vi "HFRR ADV v04 new software.vi"() -> ()   [LabVIEW 2025] (continued)
        n807 = local write "CAMERA ROI MAX TEMP"(TRUE ("CAMERA ROI MAX TEMP")) -> ()
      }
      frame "About" {
        n808 = local read "LIVE FEED MIN TEMP"() -> (w1181:bool)
        n809 = local write "LIVE FEED MAX TEMP"(TRUE ("LIVE FEED MAX TEMP")) -> ()
        n810 = local read "CAMERA ROI MIN TEMP"() -> (w1180:bool)
        n811 = case shown="True" w1181 {
          selector: w1181 -> [_ w1188]
          frame False {
          }
          frame True {
            n812 = Not(x=w1188) -> (.not. x?=w1187:bool)
            n813 = local write "LIVE FEED MIN TEMP"(w1187) -> ()
            n814 = call "CAMERA LIVE FEED FGV.vi"("Enum - Menu"=CAMERA_LIVE_FEED_ENUM."CAMERA MINIMIZE") -> ()  [unwired: 9 in, 2 out]
          }
        }
        n815 = case shown="True" w1180 {
          selector: w1180 -> [_ w1185]
          frame False {
          }
          frame True {
            n816 = Not(x=w1185) -> (.not. x?=w1184:bool)
            n817 = local write "CAMERA ROI MIN TEMP"(w1184) -> ()
            n818 = call "IMAGE ANALYSIS.vi"("Enum"=POST_ANALYSIS_ENUM."MINIMIZE UI") -> ()  [unwired: 9 in, 2 out]
          }
        }
        n819 = local write "CAMERA ROI MAX TEMP"(TRUE ("CAMERA ROI MIN TEMP")) -> ()
      }
      frame "Advance" {
        n820 = local read "LIVE FEED MIN TEMP"() -> (w1191:bool)
        n821 = local write "LIVE FEED MAX TEMP"(TRUE ("LIVE FEED MAX TEMP")) -> ()
        n822 = local read "CAMERA ROI MIN TEMP"() -> (w1189:bool)
        n823 = case shown="True" w1191 {
          selector: w1191 -> [_ w1198]
          frame False {
          }
          frame True {
            n824 = Not(x=w1198) -> (.not. x?=w1197:bool)
            n825 = local write "LIVE FEED MIN TEMP"(w1197) -> ()
            n826 = call "CAMERA LIVE FEED FGV.vi"("Enum - Menu"=CAMERA_LIVE_FEED_ENUM."CAMERA MINIMIZE") -> ()  [unwired: 9 in, 2 out]
          }
        }
        n827 = local write "CAMERA ROI MAX TEMP"(TRUE ("CAMERA ROI MAX TEMP")) -> ()
        n828 = case shown="True" w1189 {
          selector: w1189 -> [_ w1195]
          frame False {
          }
          frame True {
            n829 = Not(x=w1195) -> (.not. x?=w1194:bool)
            n830 = local write "CAMERA ROI MIN TEMP"(w1194) -> ()
            n831 = call "IMAGE ANALYSIS.vi"("Enum"=POST_ANALYSIS_ENUM."MINIMIZE UI") -> ()  [unwired: 9 in, 2 out]
          }
        }
      }
      frame "Mooha" {
        n832 = local read "LIVE FEED MIN TEMP"() -> (w1201:bool)
        n833 = local write "LIVE FEED MAX TEMP"(TRUE ("LIVE FEED MAX TEMP")) -> ()
        n834 = local read "CAMERA ROI MIN TEMP"() -> (w1199:bool)
        n835 = case shown="True" w1201 {
          selector: w1201 -> [_ w1208]
          frame False {
          }
          frame True {
            n836 = Not(x=w1208) -> (.not. x?=w1207:bool)
            n837 = local write "LIVE FEED MIN TEMP"(w1207) -> ()
            n838 = call "CAMERA LIVE FEED FGV.vi"("Enum - Menu"=CAMERA_LIVE_FEED_ENUM."CAMERA MINIMIZE") -> ()  [unwired: 9 in, 2 out]
          }
        }
        n839 = local write "CAMERA ROI MAX TEMP"(TRUE ("CAMERA ROI MAX TEMP")) -> ()
        n840 = case shown="True" w1199 {
          selector: w1199 -> [_ w1205]
          frame False {
          }
          frame True {
            n841 = Not(x=w1205) -> (.not. x?=w1204:bool)
            n842 = local write "CAMERA ROI MIN TEMP"(w1204) -> ()
            n843 = call "IMAGE ANALYSIS.vi"("Enum"=POST_ANALYSIS_ENUM."MINIMIZE UI") -> ()  [unwired: 9 in, 2 out]
          }
        }
      }
    }
    n844 = local read "Auto Start Test"() -> (w950:bool)
    n845 = case shown="True" "sign in temp" {
      frame False {
      }
      frame True {
        w987 = 1 ("y")
        n846 = local read "USERNAME"() -> (w993:string)
        n847 = local read "USER ID"() -> (w990:string)
        n848 = call <vilib>:"Trim Whitespace.vi"("string"=w993) -> ("trimmed string"=w992:string)  [unwired: 1 in]
        n849 = call <vilib>:"Trim Whitespace.vi"("string"=w990) -> ("trimmed string"=w991:string)  [unwired: 1 in]
        n850 = String Length(string=w992) -> (length=w989:i32)
        n851 = String Length(string=w991) -> (length=w988:i32)
        n852 = Greater?(x=w989, y=w987) -> (0:w986:bool)
        n853 = Greater?(x=w988, y=w987) -> (0:w985:bool)
        n854 = And(x=w986, y=w985) -> (x .and. y?=w984:bool)
        n855 = case shown="True" w984 {
          frame False {
            n856 = property on="Sign In" class="Bool (strict)"("DisabledEnum"=T13."Disabled" ("Disabled")) -> ()  [unwired: 2 in, 2 out]
          }
          frame True {
            n857 = property on="Sign In" class="Bool (strict)"("DisabledEnum"=T13."Enabled" ("Disabled")) -> ()  [unwired: 2 in, 2 out]
          }
        }
      }
    }
    n858 = local read "Air Temperature"() -> (w967:bool)
    n859 = local read "Coefficient Of Friction"() -> (w968:bool)
    n860 = case shown="False" w950 {
      frame False {
        n861 = local read "Auto stop temp"() -> (w981:bool)
        n862 = case shown="True" w981 {
          frame False {
          }
          frame True {
            n863 = local write "Auto Start Temp"(FALSE ("Auto Start Temp")) -> ()
          }
        }
      }
      frame True {
        "Auto stop temp" <- TRUE ("Auto stop temp")
      }
    }
    n864 = local read "Humidity"() -> (w966:bool)
    n865 = case shown="\"HOME\"" w978 {
      frame "HOME" {
        n866 = local write "main tab sub"(enum32{"Page 1", "Page 2"}."Page 1" ("main tab sub")) -> ()
      }
      frame Default {
        n867 = local write "main tab sub"(enum32{"Page 1", "Page 2"}."Page 2" ("main tab sub")) -> ()
      }
    }
    n868 = case shown="True" w977 {
      selector: w977 -> [_ w1313]
      frame False {
      }
      frame True {
        n869 = Not(x=w1313) -> (.not. x?=w1312:bool)
        n870 = local write "Sign In"(w1312) -> ()
        n871 = local write "Main Dashboard Buttons"(T1."Test Setup" ("Main Dashboard Buttons")) -> ()
      }
    }
    n872 = case shown="\"Numeric Display\", Default" "Num/Graph" {
      frame "Numeric Display", Default {
        n873 = property on="Single/Multiple" class="RadioBtnsControl (strict)"("Visible"=FALSE) -> ()  [unwired: 2 in, 2 out]
        n874 = property on="Single - Graph" class="Ring (strict)"("Visible"=FALSE) -> ()  [unwired: 2 in, 2 out]
        n875 = local write "Main Tab Display"(T4."Dashboard 1" ("Main Tab Display")) -> ()
      }
      frame "Graph Display" {
        n876 = property on="Single/Multiple" class="RadioBtnsControl (strict)"("Visible"=TRUE) -> ()  [unwired: 2 in, 2 out]
        n877 = case shown="\"Multiple\"" "Single/Multiple" {
          frame "Single ", Default {
            n878 = property on="Single - Graph" class="Ring (strict)"("Visible"=TRUE) -> ()  [unwired: 2 in, 2 out]
            n879 = local write "Main Tab Display"(T4."Dashboard 3" ("Main Tab Display")) -> ()
          }
          frame "Multiple" {
            n880 = property on="Single - Graph" class="Ring (strict)"("Visible"=FALSE) -> ()  [unwired: 2 in, 2 out]
            n881 = local write "Main Tab Display"(T4."Dashboard 2" ("Main Tab Display")) -> ()
          }
        }
      }
    }
    n882 = local read "Stroke"() -> (w965:bool)
    n883 = local read "USERNAME"() -> (w971:string)
    n884 = local read "USER ID"() -> (w970:string)
    n885 = case shown="True" w968 {
      selector: w968 -> [_ w1248]
      frame False {
      }
      frame True {
        n886 = Not(x=w1248) -> (.not. x?=w1247:bool)
        n887 = local write "Coefficient Of Friction"(w1247) -> ()
        n888 = local write "Tab Control 2"(T6."Coefficient Of Friction" ("Tab Control 2")) -> ()
      }
    }
    n889 = case shown="True" w967 {
      selector: w967 -> [_ w1245]
      frame False {
      }
      frame True {
        n890 = Not(x=w1245) -> (.not. x?=w1243:bool)
        n891 = local write "Air Temperature"(w1243) -> ()
        n892 = local write "Tab Control 2"(T6."Air Temperature" ("Tab Control 2")) -> ()
      }
    }
    n893 = local write "Operator ID"(w970) -> ()
    n894 = case shown="True" w965 {
      selector: w965 -> [_ w1239]
      frame False {
      }
      frame True {
        n895 = Not(x=w1239) -> (.not. x?=w1237:bool)
        n896 = local write "Stroke"(w1237) -> ()
        n897 = local write "Tab Control 2"(T6."Stroke" ("Tab Control 2")) -> ()
      }
    }
    n898 = local write "tested by"(w971) -> ()
    n899 = case shown="True" w966 {
      selector: w966 -> [_ w1242]
      frame False {
      }
      frame True {
        n900 = Not(x=w1242) -> (.not. x?=w1240:bool)
        n901 = local write "Humidity"(w1240) -> ()
        n902 = local write "Tab Control 2"(T6."Humidity" ("Tab Control 2")) -> ()
      }
    }
    n903 = case shown="\"Advance\"" "Main Dashboard Buttons" {
      tunnel: [T2."HOME" ("Main Tab") T2."Test Setup" ("Main Tab") T2."Acquire" ("Main Tab") T2."Adv Scar" ("Main Tab") T2."Adv Scar Report" ("Main Tab") T2."Compare Files" ("Main Tab") T2."About" ("Main Tab") T2."Advance" ("Main Tab")] -> w975
      frame "Home", Default {
      }
      frame "Test Setup" {
      }
      frame "Dashboard" {
      }
      frame "Imaging" {
      }
      frame "Report" {
      }
      frame "Analysis" {
      }
      frame "About" {
      }
      frame "Advance" {
      }
    }
    n904 = Wait (ms)(milliseconds to wait=u32 100) -> ()  [unwired: 1 out]
    n905 = local read "Main Tab Display"() -> (w969:T4)
    n906 = local write "Main Tab"(w975) -> ()
    n907 = case shown="\"Dashboard 3\"" w969 {
      frame "Dashboard 1", Default {
        n908 = property on="Reset Graph" class="Bool (strict)"("Visible"=FALSE) -> ()  [unwired: 2 in, 2 out]
      }
      frame "Dashboard 2" {
        n909 = property on="Reset Graph" class="Bool (strict)"("Visible"=TRUE) -> ()  [unwired: 2 in, 2 out]
      }
      frame "Dashboard 3" {
        n910 = property on="Reset Graph" class="Bool (strict)"("Visible"=TRUE) -> ()  [unwired: 2 in, 2 out]
      }
    }
    n911 = local read "SCAR MEASURMENT"() -> (w957:enum32{"Auto Scar", "Manual Scar"})
    n912 = local read "Humidity"() -> (w972:bool)
    n913 = local read "Cap Live Image"() -> (w954:bool)
    n914 = local read "Sample Temperature"() -> (w964:bool)
    n915 = local read "Air Temp vs Humidity"() -> (w962:bool)
    n916 = local read "Frequency"() -> (w963:bool)
    n917 = case shown="False" w972 {
      frame False {
        n918 = local write "Humidity On Command"(TRUE ("Humidity On Command")) -> ()
        n919 = case shown="True" "Humidity Off Command" {
          selector: "Humidity Off Command" -> [_ w1255]
          frame False {
          }
          frame True {
            n920 = stacked-sequence {
              frame #0 {
                n921 = local read "WriteHumidity"() -> (w1257:string[])
                n922 = Insert Into Array(array=w1257, new element="R;1" ("new element/subarray")) -> (w1258:string[])  [unwired: 1 in]
                n923 = local write "WriteHumidity"(w1258) -> ()
              }
              frame #1 {
                n924 = Wait (ms)(milliseconds to wait=u32 2000) -> ()  [unwired: 1 out]
              }
              frame #2 {
                n925 = local read "EVENT LOG"() -> (w1264:string)
                n926 = local read "WriteHumidity"() -> (w1261:string[])
                n927 = call "Event Log.vi"("Content"="Humidity Control Off" ("string"), "EVENT LOG"=w1264) -> ("EVENT LOG"=w1265:string)  [unwired: 8 in, 1 out]
                n928 = local write "EVENT LOG"(w1265) -> ()
                n929 = Insert Into Array(array=w1261, new element="R;1" ("new element/subarray")) -> (w1262:string[])  [unwired: 1 in]
                n930 = local write "WriteHumidity"(w1262) -> ()
              }
            }
            n931 = Not(x=w1255) -> (.not. x?=w1254:bool)
            n932 = local write "Humidity Off Command"(w1254) -> ()
          }
        }
      }
      frame True {
        n933 = local write "Humidity Off Command"(TRUE ("Humidity Off Command")) -> ()
        n934 = case shown="False" "Humidity On Command" {
          selector: "Humidity On Command" -> [_ w1269]
          frame False {
          }
          frame True {
            n935 = stacked-sequence {
              frame #0 {
                n936 = local read "Set Rh"() -> (w1275:dbl)
                n937 = Number To Fractional String(number=w1275, precision (6)=i16 2) -> (F-format string=w1276:string)  [unwired: 2 in]
                n938 = local read "WriteHumidity"() -> (w1273:string[])
                n939 = Concatenate Strings("M;" ("new element/subarray"), w1276) -> (w1274:string)
                n940 = Insert Into Array(array=w1273, new element=w1274) -> (w1272:string[])  [unwired: 1 in]
                n941 = local write "WriteHumidity"(w1272) -> ()
              }
              frame #1 {
                n942 = Wait (ms)(milliseconds to wait=u32 1500) -> ()  [unwired: 1 out]
              }
              frame #2 {
                (unwired) "% RH" ("string")
                (unwired) i16 2 ("precision (6)")
                (unwired) "M;" ("new element/subarray")
                n943 = local read "Set Rh"() -> (w1283:dbl)
                n944 = Number To Fractional String(number=w1283, precision (6)=i16 2) -> (F-format string=w1280:string)  [unwired: 2 in]
                n945 = local read "WriteHumidity"() -> (w1285:string[])
                n946 = Concatenate Strings("M;" ("new element/subarray"), w1280) -> (w1284:string)
                n947 = Concatenate Strings("Humidity Set to : " ("string"), w1280, "% RH" ("string")) -> (w1278:string)
                n948 = Insert Into Array(array=w1285, new element=w1284) -> (w1286:string[])  [unwired: 1 in]
                n949 = disable-structure shown="Enabled" {
                  frame Enabled {
                    n950 = local read "EVENT LOG"() -> (w1289:string)
                    n951 = call "Event Log.vi"("Content"="Humidity Control On", "EVENT LOG"=w1289) -> ("EVENT LOG"=w1290:string)  [unwired: 8 in, 1 out]
                    n952 = local write "EVENT LOG"(w1290) -> ()
                  }
                  frame Disabled {
                  }
                }
                n953 = disable-structure shown="Enabled" {
                  disable-tunnel: w1278 -> [_ _]
                  frame Enabled {
                    n954 = local read "EVENT LOG"() -> (w1292:string)
                    n955 = call "Event Log.vi"("Content"="Humidity Control On", "EVENT LOG"=w1292) -> ("EVENT LOG"=w1293:string)  [unwired: 8 in, 1 out]
                    n956 = local write "EVENT LOG"(w1293) -> ()
                  }
                  frame Disabled {
                  }
                }
                n957 = local write "WriteHumidity"(w1286) -> ()
              }
            }
            n958 = Not(x=w1269) -> (.not. x?=w1268:bool)
            n959 = local write "Humidity On Command"(w1268) -> ()
          }
        }
      }
    }
    n960 = Equal?(x=w957, y=enum32{"Auto Scar", "Manual Scar"}."Auto Scar" ("SCAR MEASURMENT")) -> (x = y?=w953:bool)
    n961 = local read "TEST STANDARD"() -> (w960:T3)
    n962 = And(x=w954, y=w953) -> (x .and. y?=w955:bool)
    n963 = case shown="True" w955 {
      selector: w955 -> [_ w1054]
      tunnel: errorcluster {"status"=FALSE, "code"=0, "source"=""} ("error in (no error) 3") -> [_ w1055]
      frame False {
      }
      frame True {
        n964 = stacked-sequence {
          tunnel: w1055 -> [_ _ _ _ _ _ _ w1103]
          tunnel: w1054 -> [_ _ _ _ _ w1084 _ _]
          frame #0 {
            n965 = call "CAMERA LIVE FEED FGV.vi"("Enum - Menu"=CAMERA_LIVE_FEED_ENUM."CAMERA MINIMIZE") -> ()  [unwired: 9 in, 2 out]
          }
          frame #1 {
            n966 = property on="Auto Scar Check  2" class="Clust (strict)"("Visible"=TRUE) -> ()  [unwired: 2 in, 2 out]
          }
          frame #2 {
            n967 = String To Path(string="C:\\LAB-IQ\\Image Calibrate v01.dcf") -> (path=w1060:path)
            n968 = Open/Create/Replace File ("Open File")(file path (use dialog)=w1060) -> (refnum out=w1061:refnum<file>)  [unwired: 5 in, 2 out]
            n969 = for {
              N: 4 -> [_]
              tunnel: w1061 -> [w1067]
              i -> [w1063]
              n970 = Read from Text File ("Read File")(file (use dialog)=w1067) -> (text=w1068:string)  [unwired: 3 in, 3 out]
              n971 = String Subset(string=w1068, offset (0)=6, length (rest)=10 ("length (rest)")) -> (substring=w1064:string)
              n972 = Fract/Exp String To Number(string=w1064) -> (number=w1062:dbl)  [unwired: 3 in, 1 out]
              n973 = case shown="0" w1063 {
                tunnel: w1062 -> [w1069 w1070 _ w1071 _]
                frame 0 {
                  "5x Gain" <- w1069
                }
                frame 1 {
                  "10x Gain" <- w1070
                }
                frame 2 {
                }
                frame 3 {
                  "100x gain" <- w1071
                }
                frame 4, Default {
                }
              }
            }
          }
          frame #3 {
            n974 = local read "FILE 3"() -> (w1077:string)
            n975 = call <vilib>:"Trim Whitespace.vi"("string"="C:\\LAB-IQ\\images\\") -> ("trimmed string"=w1079:string)  [unwired: 1 in]
            n976 = String To Path(string=w1079) -> (path=w1078:path)
            n977 = Concatenate Strings(w1077, ".png" ("string")) -> (w1076:string)
            n978 = Build Path(base path=w1078, name or relative path=w1076) -> (appended path=w1074:path)
            "Image path" <- w1074
            n979 = Path To String(path=w1074) -> (string=w1073:string)
            n980 = call "CAMERA LIVE FEED FGV.vi"("Enum - Menu"=CAMERA_LIVE_FEED_ENUM."CAMERA SAVE", "Image Path"=w1073) -> ()  [unwired: 8 in, 2 out]
          }
          frame #4 {
            n981 = One Button Dialog(message="Image saved successfully") -> ()  [unwired: 1 in, 1 out]
          }
          frame #5 {
            n982 = local read "TEST STANDARD"() -> (w1083:T3)
            n983 = local read "Magnification len live scar"() -> (w1095:string)
            n984 = Not(x=w1084) -> (.not. x?=w1085:bool)
            n985 = local write "Cap Live Image"(w1085) -> ()
            n986 = case shown="\"ISO 12156\"" w1083 {
              tunnel: ["ASTM D6079" "ISO 12156"] -> w1082
              frame "ASTM D6079", Default {
              }
              frame "ISO 12156" {
              }
            }
            n987 = case shown="\"5x\", Default" w1095 {
              tunnel: [w1098 w1099] -> w1094
              frame "5x", Default {
                n988 = local read "5x Gain"() -> (w1098:dbl)
              }
              frame "10x" {
                # "5x"
                n989 = local read "10x Gain"() -> (w1099:dbl)
              }
            }
            n990 = local read "Image path"() -> (w1093:path)
            n991 = local read "FILE 3"() -> (w1086:string)
            n992 = call "EDGE DETCTION.vi"("GAIN VALUE"=w1094, "Image Path"=w1093) -> ("error out"=w1092:errorcluster, "return value"=w1091:cluster{string, string, dbl, dbl, dbl})  [unwired: 8 in]
            n993 = Bundle By Name(cluster=T18 {"File Name"="", "Test Method"="", "Operator"="", "Fuel Description"="", "Date and time"=""} ("Main Ref"), "File Name"=w1086, "Test Method"=w1082) -> (w1087:T18)
            n994 = call "duf file read.vi"("error in (no error)"=w1092, "Main Ref"=w1087) -> ("error out"=w1090:errorcluster, "Main Ref 2"=w1088:T18)  [unwired: 8 in]
            n995 = call "EDGE DETECTION REPORT.vi"("error in (no error)"=w1090, "return value 2"=w1091, "Main Ref"=w1088) -> ()  [unwired: 8 in, 1 out]
          }
          frame #6 {
            n996 = property on="Auto Scar Check  2" class="Clust (strict)"("Visible"=FALSE) -> ()  [unwired: 2 in, 2 out]
          }
          frame #7 {
            n997 = call "CAMERA LIVE FEED FGV.vi"("Enum - Menu"=CAMERA_LIVE_FEED_ENUM."CAMERA MINIMIZE", "error in (no error)"=w1103) -> ()  [unwired: 8 in, 2 out]
            n998 = local write "Main Dashboard Buttons"(T1."Home" ("Main Dashboard Buttons")) -> ()
            n999 = local write "Main Tab"(T2."HOME" ("Main Tab")) -> ()
          }
        }
      }
    }
    n1000 = local read "Heater Button"() -> (w961:bool)
    n1001 = case shown="True" w963 {
      selector: w963 -> [_ w1233]
      frame False {
      }
      frame True {
        n1002 = Not(x=w1233) -> (.not. x?=w1231:bool)
        n1003 = local write "Frequency"(w1231) -> ()
        n1004 = local write "Tab Control 2"(T6."Frequency" ("Tab Control 2")) -> ()
      }
    }
    n1005 = case shown="True" w962 {
      selector: w962 -> [_ w1230]
      frame False {
      }
      frame True {
        n1006 = Not(x=w1230) -> (.not. x?=w1228:bool)
        n1007 = local write "Air Temp vs Humidity"(w1228) -> ()
        n1008 = local write "Tab Control 2"(T6."Air Temp vs Rh" ("Tab Control 2")) -> ()
      }
    }
    n1009 = case shown="True" w964 {
      selector: w964 -> [_ w1236]
      frame False {
      }
      frame True {
        n1010 = Not(x=w1236) -> (.not. x?=w1234:bool)
        n1011 = local write "Sample Temperature"(w1234) -> ()
        n1012 = local write "Tab Control 2"(T6."Sample Temperature" ("Tab Control 2")) -> ()
      }
    }
    n1013 = case shown="\"Custom\"" w960 {
      frame "ASTM D6079", Default {
        w1209 = "ASTM D6079 TEST CONDITIONS" ("Standard 2")
        n1014 = local write "Standard 2"(w1209) -> ()
        n1015 = local write "Standard"(w1209) -> ()
      }
      frame "ISO 12156" {
        w1210 = "ISO 12156 TEST CONDITIONS" ("Standard 2")
        n1016 = local write "Standard 2"(w1210) -> ()
        n1017 = local write "Standard"(w1210) -> ()
      }
      frame "CEC F-096-A-06" {
        w1211 = "CEC F-096-A-06 TEST CONDITIONS" ("Standard 2")
        n1018 = local write "Standard 2"(w1211) -> ()
        n1019 = local write "Standard"(w1211) -> ()
      }
      frame "Custom" {
        w1212 = "CUSTOM TEST CONDITIONS" ("Standard 2")
        n1020 = local write "Standard 2"(w1212) -> ()
        n1021 = local write "Standard"(w1212) -> ()
      }
    }
    n1022 = case shown="True" w961 {
      frame False {
        n1023 = local write "Temperature On Command"(TRUE ("Temperature On Command")) -> ()
        n1024 = case shown="True" "Temperature Off Command" {
          selector: "Temperature Off Command" -> [_ w1216]
          frame False {
          }
          frame True {
            n1025 = Not(x=w1216) -> (.not. x?=w1215:bool)
            n1026 = local read "EVENT LOG"() -> (w1219:string)
            n1027 = local write "Temperature Off Command"(w1215) -> ()
            n1028 = call "Event Log.vi"("Content"="Heater Off", "EVENT LOG"=w1219) -> ("EVENT LOG"=w1218:string)  [unwired: 8 in, 1 out]
            n1029 = local write "EVENT LOG"(w1218) -> ()
          }
        }
      }
      frame True {
        n1030 = local write "Temperature Off Command"(TRUE ("Temperature Off Command")) -> ()
        n1031 = case shown="True" "Temperature On Command" {
          selector: "Temperature On Command" -> [_ w1223]
          frame False {
          }
          frame True {
            n1032 = Not(x=w1223) -> (.not. x?=w1222:bool)
            n1033 = local write "Temperature On Command"(w1222) -> ()
            n1034 = disable-structure shown="Enabled" {
              disable-tunnel: "Heater On" -> [w1225 _]
              frame Enabled {
                n1035 = local read "EVENT LOG"() -> (w1226:string)
                n1036 = call "Event Log.vi"("Content"=w1225, "EVENT LOG"=w1226) -> ("EVENT LOG"=w1227:string)  [unwired: 8 in, 1 out]
                n1037 = local write "EVENT LOG"(w1227) -> ()
              }
              frame Disabled {
              }
            }
          }
        }
      }
    }
    n1038 = local read "Main Tab"() -> (w952:T2)
    n1039 = case shown="\"About\"" w952 {
      frame "HOME", Default {
        w998 = T13."Enabled" ("Disabled")
        n1040 = local read "Service Password enable"() -> (w997:bool)
        n1041 = property on="Imaging" class="Bool (strict)"("DisabledEnum"=w998) -> ()  [unwired: 2 in, 2 out]
        n1042 = property on="Dashboard" class="Bool (strict)"("DisabledEnum"=w998) -> ()  [unwired: 2 in, 2 out]
        n1043 = property on="Test Setup" class="Bool (strict)"("DisabledEnum"=w998) -> ()  [unwired: 2 in, 2 out]
        n1044 = property on="Analysis" class="Bool (strict)"("DisabledEnum"=w998) -> ()  [unwired: 2 in, 2 out]
        n1045 = property on="Home" class="Bool (strict)"("DisabledEnum"=w998) -> ()  [unwired: 2 in, 2 out]
        n1046 = property on="Report" class="Bool (strict)"("DisabledEnum"=w998) -> ()  [unwired: 2 in, 2 out]
        n1047 = property on="Main Dashboard Buttons" class="RadioBtnsControl (strict)"("DisabledEnum"=w998) -> ()  [unwired: 2 in, 2 out]
        n1048 = case shown="True" w997 {
          tunnel: [T13."Disabled" ("Disabled") T13."Enabled" ("Disabled")] -> w996
          frame False {
          }
          frame True {
          }
        }
        n1049 = property on="About" class="Bool (strict)"("DisabledEnum"=w996) -> ()  [unwired: 2 in, 2 out]
      }
      frame "Test Setup" {
        w1003 = T13."Enabled" ("Disabled")
        n1050 = local read "Service Password enable"() -> (w1002:bool)
        n1051 = property on="Dashboard" class="Bool (strict)"("DisabledEnum"=T13."Disabled" ("Disabled")) -> ()  [unwired: 2 in, 2 out]
        n1052 = property on="Imaging" class="Bool (strict)"("DisabledEnum"=w1003) -> ()  [unwired: 2 in, 2 out]
        n1053 = property on="Analysis" class="Bool (strict)"("DisabledEnum"=w1003) -> ()  [unwired: 2 in, 2 out]
        n1054 = property on="Home" class="Bool (strict)"("DisabledEnum"=w1003) -> ()  [unwired: 2 in, 2 out]
        n1055 = property on="Report" class="Bool (strict)"("DisabledEnum"=w1003) -> ()  [unwired: 2 in, 2 out]
        n1056 = property on="Test Setup" class="Bool (strict)"("DisabledEnum"=w1003) -> ()  [unwired: 2 in, 2 out]
        n1057 = case shown="True" w1002 {
          tunnel: [T13."Disabled" ("Disabled") T13."Enabled" ("Disabled")] -> w1001
          frame False {
          }
          frame True {
          }
        }
        n1058 = property on="About" class="Bool (strict)"("DisabledEnum"=w1001) -> ()  [unwired: 2 in, 2 out]
      }
      frame "Adv Scar" {
        w1010 = T13."Enabled" ("Disabled")
        n1059 = property on="Dashboard" class="Bool (strict)"("DisabledEnum"=T13."Disabled" ("Disabled")) -> ()  [unwired: 2 in, 2 out]
        n1060 = property on="Imaging" class="Bool (strict)"("DisabledEnum"=w1010) -> ()  [unwired: 2 in, 2 out]
        n1061 = property on="Analysis" class="Bool (strict)"("DisabledEnum"=w1010) -> ()  [unwired: 2 in, 2 out]
        n1062 = property on="Home" class="Bool (strict)"("DisabledEnum"=w1010) -> ()  [unwired: 2 in, 2 out]
        n1063 = property on="Report" class="Bool (strict)"("DisabledEnum"=w1010) -> ()  [unwired: 2 in, 2 out]
        n1064 = property on="Test Setup" class="Bool (strict)"("DisabledEnum"=w1010) -> ()  [unwired: 2 in, 2 out]
        n1065 = local read "Service Password enable"() -> (w1008:bool)
        n1066 = case shown="True" w1008 {
          tunnel: [T13."Disabled" ("Disabled") T13."Enabled" ("Disabled")] -> w1007
          frame False {
          }
          frame True {
          }
        }
        n1067 = property on="About" class="Bool (strict)"("DisabledEnum"=w1007) -> ()  [unwired: 2 in, 2 out]
      }
      frame "Adv Scar Report" {
        w1015 = T13."Enabled" ("Disabled")
        n1068 = property on="Dashboard" class="Bool (strict)"("DisabledEnum"=T13."Disabled" ("Disabled")) -> ()  [unwired: 2 in, 2 out]
        n1069 = property on="Imaging" class="Bool (strict)"("DisabledEnum"=w1015) -> ()  [unwired: 2 in, 2 out]
        n1070 = property on="Analysis" class="Bool (strict)"("DisabledEnum"=w1015) -> ()  [unwired: 2 in, 2 out]
        n1071 = property on="Home" class="Bool (strict)"("DisabledEnum"=w1015) -> ()  [unwired: 2 in, 2 out]
        n1072 = property on="Report" class="Bool (strict)"("DisabledEnum"=w1015) -> ()  [unwired: 2 in, 2 out]
        n1073 = property on="Test Setup" class="Bool (strict)"("DisabledEnum"=w1015) -> ()  [unwired: 2 in, 2 out]
        n1074 = local read "Service Password enable"() -> (w1014:bool)
        n1075 = case shown="True" w1014 {
          tunnel: [T13."Disabled" ("Disabled") T13."Enabled" ("Disabled")] -> w1013
          frame False {
          }
          frame True {
          }
        }
        n1076 = property on="About" class="Bool (strict)"("DisabledEnum"=w1013) -> ()  [unwired: 2 in, 2 out]
      }
      frame "Compare Files" {
        w1021 = T13."Enabled" ("Disabled")
        n1077 = local read "Service Password enable"() -> (w1020:bool)
        n1078 = property on="Dashboard" class="Bool (strict)"("DisabledEnum"=T13."Disabled" ("Disabled")) -> ()  [unwired: 2 in, 2 out]
        n1079 = property on="Imaging" class="Bool (strict)"("DisabledEnum"=w1021) -> ()  [unwired: 2 in, 2 out]
        n1080 = property on="Analysis" class="Bool (strict)"("DisabledEnum"=w1021) -> ()  [unwired: 2 in, 2 out]
        n1081 = property on="Home" class="Bool (strict)"("DisabledEnum"=w1021) -> ()  [unwired: 2 in, 2 out]
        n1082 = property on="Report" class="Bool (strict)"("DisabledEnum"=w1021) -> ()  [unwired: 2 in, 2 out]
        n1083 = property on="Test Setup" class="Bool (strict)"("DisabledEnum"=w1021) -> ()  [unwired: 2 in, 2 out]
        n1084 = case shown="True" w1020 {
          tunnel: [T13."Disabled" ("Disabled") T13."Enabled" ("Disabled")] -> w1019
          frame False {
          }
          frame True {
          }
        }
        n1085 = property on="About" class="Bool (strict)"("DisabledEnum"=w1019) -> ()  [unwired: 2 in, 2 out]
      }
      frame "Acquire" {
        n1086 = local read "Service Password enable"() -> (w1025:bool)
        n1087 = property on="Test Setup" class="Bool (strict)"("DisabledEnum"=T13."Disabled" ("Disabled")) -> ()  [unwired: 2 in, 2 out]
        n1088 = local read "Auto Start Test"() -> (w1027:bool)
        n1089 = local read "RUN"() -> (w1029:bool)
        n1090 = case shown="True" w1025 {
          tunnel: [T13."Disabled" ("Disabled") T13."Enabled" ("Disabled")] -> w1026
          frame False {
          }
          frame True {
          }
        }
        n1091 = Or(x=w1029, y=w1027) -> (x .or. y?=w1028:bool)
        n1092 = case shown="True" w1028 {
          tunnel: [T13."Enabled" ("Disabled") T13."Disabled" ("Disabled")] -> w1031
          frame False {
          }
          frame True {
          }
        }
        n1093 = property on="About" class="Bool (strict)"("DisabledEnum"=w1026) -> ()  [unwired: 2 in, 2 out]
        n1094 = property on="Imaging" class="Bool (strict)"("DisabledEnum"=w1031) -> ()  [unwired: 2 in, 2 out]
        n1095 = property on="Dashboard" class="Bool (strict)"("DisabledEnum"=w1031) -> ()  [unwired: 2 in, 2 out]
        n1096 = property on="Analysis" class="Bool (strict)"("DisabledEnum"=w1031) -> ()  [unwired: 2 in, 2 out]
        n1097 = property on="Home" class="Bool (strict)"("DisabledEnum"=w1031) -> ()  [unwired: 2 in, 2 out]
        n1098 = property on="Report" class="Bool (strict)"("DisabledEnum"=w1031) -> ()  [unwired: 2 in, 2 out]
      }
      frame "About" {
        n1099 = local read "FILE"() -> (w1044:string)
        n1100 = local read "TEST FILE NAM,E SAVED"() -> (w1037:bool)
        n1101 = call <vilib>:"Trim Whitespace.vi"("string"=w1044) -> ("trimmed string"=w1043:string)  [unwired: 1 in]
        n1102 = local read "Auto Start Test"() -> (w1047:bool)
        n1103 = String Length(string=w1043) -> (length=w1042:i32)
        n1104 = Greater?(x=w1042, y=1) -> (0:w1039:bool)
        n1105 = And(x=w1039, y=w1037) -> (x .and. y?=w1038:bool)
        n1106 = local read "RUN"() -> (w1049:bool)
        n1107 = case shown="True" w1038 {
          tunnel: [T13."Disabled" ("Disabled") T13."Enabled" ("Disabled")] -> w1040
          frame False {
          }
          frame True {
          }
        }
        n1108 = Or(x=w1049, y=w1047) -> (x .or. y?=w1048:bool)
        n1109 = property on="About" class="Bool (strict)"("DisabledEnum"=T13."Enabled" ("Disabled")) -> ()  [unwired: 2 in, 2 out]
        n1110 = case shown="False" w1048 {
          tunnel: [T13."Enabled" ("Disabled") T13."Disabled" ("Disabled")] -> w1046
          frame False {
          }
          frame True {
          }
        }
        n1111 = property on="Dashboard" class="Bool (strict)"("DisabledEnum"=w1040) -> ()  [unwired: 2 in, 2 out]
        n1112 = property on="Test Setup" class="Bool (strict)"("DisabledEnum"=T13."Disabled" ("Disabled")) -> ()  [unwired: 2 in, 2 out]
        n1113 = property on="Imaging" class="Bool (strict)"("DisabledEnum"=w1046) -> ()  [unwired: 2 in, 2 out]
        n1114 = property on="Analysis" class="Bool (strict)"("DisabledEnum"=w1046) -> ()  [unwired: 2 in, 2 out]
        n1115 = property on="Home" class="Bool (strict)"("DisabledEnum"=w1046) -> ()  [unwired: 2 in, 2 out]
        n1116 = property on="Report" class="Bool (strict)"("DisabledEnum"=w1046) -> ()  [unwired: 2 in, 2 out]
      }
    }
    n1117 = local read "Quit"() -> (w980:bool)
    "Single" <- "Single - Graph"
  }
  n1118 = disable-structure shown="Disabled" {
    disable-tunnel: [w1317 _] -> w39
    disable-tunnel: _ -> [w1316 _]
    frame Disabled {
      n1119 = while {
        tunnel: w1316 -> [_]
        tunnel: [w1318] -> w1317
        tunnel: [w1319] -> _
        i -> [w1319]
        stop <- w1318 stop-if-true
        w1335 = u16 10 items=["1.0"=10, "1.5"=15, "2.0"=20] ("stop bits (10: 1 bit)")
        n1120 = Wait (ms)(milliseconds to wait=u32 10) -> ()  [unwired: 1 out]
        n1121 = call-poly "VISA Configure Serial Port"("VISA resource name"=refnum<visa-resource-name> "ASRL1::INSTR" ("COM PORT"), "timeout (10sec)"=u32 10, "baud rate (9600)"=u32 57600, "data bits (8)"=u16 8, "stop bits (10: 1 bit)"=w1335) -> ("VISA resource name out"=w1321:refnum<visa-resource-name>, "error out"=w1330:errorcluster)  [unwired: 9 in]
        n1122 = VISA Read(VISA resource name=w1321, byte count=u32 2 ("byte count (0)")) -> (read buffer=w1329:string)  [unwired: 1 in, 3 out]
        n1123 = String Subset(string=w1329, offset (0)=0, length (rest)=2 ("length (rest)")) -> (substring=w1328:string)
        n1124 = Match Pattern(string=w1328, regular expression="<>") -> (offset past match=w1325:i32)  [unwired: 1 in, 3 out]
        n1125 = Greater Or Equal?(x=w1325, y=0) -> (x >= y?=w1320:bool)
        n1126 = case shown="True" w1320 {
          tunnel: w1321 -> [_ w1339]
          tunnel: w1330 -> [_ w1338]
          frame False {
          }
          frame True {
            n1127 = VISA Read(VISA resource name=w1339, byte count=u32 32 ("byte count (0)"), error in (no error)=w1338) -> (read buffer=w1337:string)  [unwired: 3 out]
            n1128 = String Subset(string=w1337, offset (0)=0, length (rest)=8 ("length (rest)")) -> (substring=w1341:string)
            n1129 = String Subset(string=w1337, offset (0)=8, length (rest)=8 ("length (rest)")) -> (substring=w1342:string)
            n1130 = Decimal String To Number(string=w1342) -> (number=w1349:i32)  [unwired: 2 in, 1 out]
            n1131 = Decimal String To Number(string=w1341) -> (number=w1345:i32)  [unwired: 2 in, 1 out]
            n1132 = Divide(x=w1349, y=10000) -> ()  [unwired: 1 out]
            n1133 = Divide(x=w1345, y=1000000) -> ()  [unwired: 1 out]
          }
        }
        n1134 = local read "Quit"() -> (w1318:bool)
      }
    }
    frame Enabled {
    }
  }
  n1135 = while {
    shift-right: [w1364] -> w52
    shift-left: _ -> [w1355]
    shift-right: [w1363] -> w51
    shift-left: errorcluster {"status"=TRUE, "code"=0, "source"="Init"} ("error IO") -> [w1357]
    tunnel: [w1352] -> w42
    tunnel: [w1362] -> _
    i -> [w1362]
    stop <- w1352 stop-if-true
    n1136 = local read "Port 1a"() -> (w1358:bool)
    n1137 = local read "Port 3"() -> (w1359:bool)
    n1138 = local read "Com Port 1"() -> (w1356:refnum<visa-resource-name>)
    n1139 = Or(x=w1359, y=w1358) -> (x .or. y?=w1361:bool)
    n1140 = Unbundle(w1357) -> ("status"=→"Port 3":bool)  [unwired: 2 out]
    n1141 = Not Equal?(x=w1356, y=w1355) -> (x != y?=w1353:bool)
    n1142 = case shown="True" w1361 {
      frame False {
        w1367 = FALSE ("Visible")
        n1143 = property on="Port 1a" class="Bool (strict)"("Visible"=w1367) -> ()  [unwired: 2 in, 2 out]
        n1144 = property on="Port 3" class="Bool (strict)"("Visible"=w1367) -> ()  [unwired: 2 in, 2 out]
      }
      frame True {
        w1368 = TRUE ("Visible")
        n1145 = property on="Port 1a" class="Bool (strict)"("Visible"=w1368) -> ()  [unwired: 2 in, 2 out]
        n1146 = property on="Port 3" class="Bool (strict)"("Visible"=w1368) -> ()  [unwired: 2 in, 2 out]
      }
    }
    n1147 = Wait (ms)(milliseconds to wait=u32 10) -> ()  [unwired: 1 out]
    n1148 = case shown="True" w1353 {
      tunnel: [w1365 errorcluster {"status"=TRUE, "code"=0, "source"="Init"} ("error out")] -> w1354
      tunnel: w1357 -> [w1365 _]
      frame False {
      }
      frame True {
      }
    }
    n1149 = case shown="No Error" w1354 {
      selector: w1354 -> [w1376 w1403]
      tunnel: [w1369 w1407] -> w1364
      tunnel: [w1378 w1401] -> w1363
      tunnel: w1355 -> [w1377 w1405]
      frame No Error {
        n1150 = property class="Instr"(reference=w1377, error in=w1376) -> (reference out=w1374:refnum<visa-resource-name>, error out=w1375:errorcluster, "Serial Settings:Number of Bytes at Serial Port"=w1370:u32)
        n1151 = Greater?(x=w1370, y=u32 5) -> (0:w1372:bool)
        n1152 = Not(x=w1372) -> (.not. x?=→"Port 1a":bool)
        n1153 = while {
          tunnel: [w1396] -> w1378
          tunnel: [w1395] -> w1379
          tunnel: w1375 -> [w1394]
          tunnel: w1374 -> [w1393]
          stop <- TRUE stop-if-true
          n1154 = property class="Instr" props=["Serial Settings:Number of Bytes at Serial Port"](reference=w1393, error in=w1394) -> (reference out=w1398:refnum<visa-resource-name>, error out=w1397:errorcluster)  [unwired: 1 out]
          n1155 = VISA Read(VISA resource name=w1398, byte count=u32 1000, error in (no error)=w1397) -> (VISA resource name out=w1395:refnum<visa-resource-name>, read buffer=w1380:string, error out=w1396:errorcluster)  [unwired: 1 out]
          "UNI READ" <- w1380
          n1156 = Spreadsheet String To Array(delimiter (Tab)=";", format string="", spreadsheet string=w1380, array type (2D Dbl)=dbl[] []) -> (array=w1390:dbl[])
          n1157 = Index Array(array=w1390) -> (element #1=→"LVDT MIN":dbl, element #2=→"LVDT MAX":dbl, element #3=→"LVDT Peak":dbl, element #4=→"pizo raw":dbl, element #5=→"Friction":dbl, element #6=→"cof 2":dbl)  [unwired: 6 in]
        }
        n1158 = VISA Flush I/O Buffer(VISA resource name=w1379) -> (VISA resource name out=w1369:refnum<visa-resource-name>)  [unwired: 2 in, 1 out]
      }
      frame Error {
        w1413 = u16 0 items=["None", "XON/XOFF", "RTS/CTS", "XON/XOFF & RTS/CTS", "DTR/DSR", "XON/XOFF & DTR/DSR"] ("flow control (0:none)  2")
        w1411 = u16 10 items=["1.0"=10, "1.5"=15, "2.0"=20] ("stop bits 2")
        w1409 = u16 0 items=["None", "Odd", "Even", "Mark", "Space"] ("parity 2")
        w1410 = u32 10000  # timeout (10sec)
        n1159 = VISA Close(VISA resource name=w1405, error in (no error)=w1403) -> (error out=w1406:errorcluster)
        n1160 = local write "Port 1a"(FALSE ("Port 1a")) -> ()
        n1161 = local read "Com Port 1"() -> (w1400:refnum<visa-resource-name>)
        n1162 = call <vilib>:"Clear Errors.vi"("error in (no error)"=w1406) -> ("error out"=w1404:errorcluster)  [unwired: 5 in, 1 out]
        n1163 = call-poly "VISA Configure Serial Port"("VISA resource name"=w1400, "timeout (10sec)"=w1410, "baud rate (9600)"=u32 250000 ("baud rate  2"), "data bits (8)"=u16 8 ("data bits  2"), "parity (0:none)"=w1409, "error in (no error)"=w1404, "stop bits (10: 1 bit)"=w1411, "flow control (0:none)"=w1413) -> ("VISA resource name out"=w1414:refnum<visa-resource-name>, "error out"=w1415:errorcluster)  [unwired: 6 in]
        n1164 = flat-sequence {
          tunnel: w1414 -> [w1417]
          tunnel: w1415 -> [w1416]
          tunnel: [w1417] -> w1407
          tunnel: [w1416] -> w1401
          frame #0 {
            n1165 = Wait (ms)(milliseconds to wait=u32 50) -> ()  [unwired: 1 out]
          }
        }
        "Residual Uno" <- ""
        "Port 1 Error" <- w1401
      }
    }
    n1166 = local read "Quit"() -> (w1352:bool)
    "Error Uno" <- w1357
  }
  n1167 = while {
    stop <- w1424 stop-if-true
    # "V0OLTAGE TO STROKE (peice vise calibration)"
    n1168 = Wait (ms)(milliseconds to wait=u32 10) -> ()  [unwired: 1 out]
    n1169 = local read "LVDT Peak"() -> (w1421:dbl)
    n1170 = formula code="// Dynamic Parameterized Linear Interpolation Node\n// Inputs: vpp_val, voltages (Array), distances (Array)\n// Outputs: stroke\n\nint i = 0;\nint segments = 11; // 12 points make 11 interpolation segments\n\n// 1. Lower Boundary Clamp\nif (vpp_val <= voltages[0]) {\n    stroke = distances[0];\n}\n// 2. Upper Boundary Clamp\nelse if (vpp_val >= voltages[segments]) {\n    stroke = distances[segments];\n}\n// 3. Dynamic Segment Search Loop\nelse {\n    stroke = distances[0]; // Fallback baseline\n    for (i = 0; i < segments; i++) {\n        if (vpp_val >= voltages[i] && vpp_val <= voltages[i+1]) {\n            // Standard linear interpolation formula using array lookups\n            stroke = distances[i] + (vpp_val - voltages[i]) * (distances[i+1] - distances[i]) / (voltages[i+1] - voltages[i]);\n            break; // Segment found, safely exit the loop\n        }\n    }\n}"("vpp_val"=w1421, "voltages"="calibration values", "distances"="STROKE") -> ("stroke"=w1420:dbl)
    n1171 = local write "measured_stroke"(w1420) -> ()
    n1172 = local read "Quit"() -> (w1424:bool)
  }
  n1173 = while {
    stop <- w1444 stop-if-true
    n1174 = call <vilib>:"High Resolution Polling Wait.vi"("seconds to wait"=0.02) -> ()  [unwired: 10 in, 1 out]
    n1175 = local read "Due read"() -> (w1442:string)
    n1176 = Spreadsheet String To Array(delimiter (Tab)=";", format string="", spreadsheet string=w1442, array type (2D Dbl)=string[] []) -> (array=w1439:string[])
    n1177 = Fract/Exp String To Number(string=w1439) -> (number=w1438:dbl[])  [unwired: 3 in, 1 out]
    n1178 = Index Array(array=w1438) -> (element #1=→"Sample Temperature":dbl, element #2=→"Target Sample Temperature":dbl, element #3=→"Current Duty Cycle":dbl, element #4=→"Ambient Temperature":dbl, element #5=→"Dac Status":dbl, element #6=→"Vpp":dbl, element #7=→"Active Error Code":dbl, element #8=→"Kp":dbl, element #9=→"Ki":dbl, element #10=→"Kd":dbl, element #11=→"SampleRaw":dbl, element #12=→"AmbRaw":dbl)  [unwired: 12 in]
    n1179 = local read "Quit"() -> (w1444:bool)
  }
  n1180 = while {
    shift-right: [w1458] -> w37
    shift-left: _ -> [w1449]
    shift-right: [w1457] -> w36
    shift-left: errorcluster {"status"=FALSE, "code"=0, "source"="Init"} ("error out") -> [w1451]
    tunnel: [w1446] -> w41
    tunnel: [w1456] -> _
    i -> [w1456]
    stop <- w1446 stop-if-true
    n1181 = local read "Com Port 2"() -> (w1450:refnum<visa-resource-name>)
    n1182 = local read "Port 2a"() -> (w1452:bool)
    n1183 = Unbundle(w1451) -> ("status"=→"Port 4":bool)  [unwired: 2 out]
    n1184 = call <vilib>:"High Resolution Polling Wait.vi"("seconds to wait"=0.02) -> ()  [unwired: 10 in, 1 out]
    n1185 = local read "Port 4"() -> (w1453:bool)
    n1186 = Not Equal?(x=w1450, y=w1449) -> (x != y?=w1448:bool)
    n1187 = Or(x=w1453, y=w1452) -> (x .or. y?=w1455:bool)
    n1188 = case shown="True" w1455 {
      frame False {
        w1461 = FALSE ("Visible")
        n1189 = property on="Port 2a" class="Bool (strict)"("Visible"=w1461) -> ()  [unwired: 2 in, 2 out]
        n1190 = property on="Port 4" class="Bool (strict)"("Visible"=w1461) -> ()  [unwired: 2 in, 2 out]
      }
      frame True {
        w1462 = TRUE ("Visible")
        n1191 = property on="Port 2a" class="Bool (strict)"("Visible"=w1462) -> ()  [unwired: 2 in, 2 out]
        n1192 = property on="Port 4" class="Bool (strict)"("Visible"=w1462) -> ()  [unwired: 2 in, 2 out]
      }
    }
    n1193 = case shown="True" w1448 {
      tunnel: [w1459 errorcluster {"status"=TRUE, "code"=0, "source"="Init"} ("error out")] -> w1447
      tunnel: w1451 -> [w1459 _]
      frame False {
      }
      frame True {
      }
    }
    n1194 = case shown="No Error" w1447 {
      selector: w1447 -> [w1473 w1504]
      tunnel: [w1466 w1509] -> w1458
      tunnel: [w1474 w1502] -> w1457
      tunnel: w1449 -> [w1476 w1507]
      frame No Error {
        n1195 = property class="Instr" props=["Serial Settings:Number of Bytes at Serial Port"](reference=w1476, error in=w1473) -> (reference out=w1467:refnum<visa-resource-name>, error out=w1472:errorcluster)  [unwired: 1 out]
        n1196 = while {
          tunnel: [w1484] -> w1468
          tunnel: [w1483] -> w1469
          tunnel: w1472 -> [w1482]
          tunnel: w1467 -> [w1481]
          tunnel: [w1480] -> _
          i -> [w1480]
          stop <- TRUE stop-if-true
          n1197 = property class="Instr" props=["Serial Settings:Number of Bytes at Serial Port"](reference=w1481, error in=w1482) -> (reference out=w1486:refnum<visa-resource-name>, error out=w1485:errorcluster)  [unwired: 1 out]
          n1198 = VISA Read(VISA resource name=w1486, byte count=u32 1000, error in (no error)=w1485) -> (VISA resource name out=w1483:refnum<visa-resource-name>, read buffer=→"Due read":string, error out=w1484:errorcluster)  [unwired: 1 out]
        }
        n1199 = local read "Command"() -> (w1464:string)
        n1200 = call <vilib>:"Trim Whitespace.vi"("string"=w1464) -> ("trimmed string"=w1463:string)  [unwired: 1 in]
        n1201 = Not Equal?(x=w1463, y="") -> (x != y?=w1470:bool)
        n1202 = case shown="True" w1470 {
          tunnel: w1469 -> [w1488 w1493]
          tunnel: [w1488 w1497] -> w1475
          tunnel: w1468 -> [w1487 w1492]
          tunnel: [w1487 w1495] -> w1474
          tunnel: w1463 -> [_ w1491]
          tunnel: [_ w1494] -> _
          frame False {
            # "DATA  WRITE LOOP"
          }
          frame True {
            n1203 = Concatenate Strings(w1491, "\r\n") -> (w1490:string)
            n1204 = VISA Write(VISA resource name=w1493, write buffer=w1490, error in (no error)=w1492) -> (VISA resource name out=w1497:refnum<visa-resource-name>, return count=w1494:u32, error out=w1496:errorcluster)
            n1205 = flat-sequence {
              tunnel: w1496 -> [w1499]
              tunnel: [w1499] -> w1495
              frame #0 {
                n1206 = local write "Command"("" ("Command")) -> ()
                n1207 = Wait (ms)(milliseconds to wait=u32 5) -> ()  [unwired: 1 out]
              }
            }
          }
        }
        n1208 = VISA Flush I/O Buffer(VISA resource name=w1475) -> (VISA resource name out=w1466:refnum<visa-resource-name>, error out=→"error out 9":errorcluster)  [unwired: 2 in]
      }
      frame Error {
        w1515 = u16 0 items=["None", "XON/XOFF", "RTS/CTS", "XON/XOFF & RTS/CTS", "DTR/DSR", "XON/XOFF & DTR/DSR"] ("flow control (0:none)  2")
        w1513 = u16 10 items=["1.0"=10, "1.5"=15, "2.0"=20] ("stop bits 2")
        w1511 = u16 0 items=["None", "Odd", "Even", "Mark", "Space"] ("parity 2")
        w1512 = u32 10000  # timeout (10sec)
        n1209 = VISA Clear(VISA resource name=w1507, error in (no error)=w1504) -> (VISA resource name out=w1506:refnum<visa-resource-name>, error out=w1505:errorcluster)
        n1210 = VISA Close(VISA resource name=w1506, error in (no error)=w1505) -> (error out=w1508:errorcluster)
        n1211 = call <vilib>:"Clear Errors.vi"("error in (no error)"=w1508) -> ()  [unwired: 5 in, 2 out]
        n1212 = local read "Com Port 2"() -> (w1501:refnum<visa-resource-name>)
        "visa due" <- w1501
        n1213 = call-poly "VISA Configure Serial Port"("VISA resource name"=w1501, "timeout (10sec)"=w1512, "baud rate (9600)"=u32 250000 ("baud rate  2"), "data bits (8)"=u16 8 ("data bits  2"), "parity (0:none)"=w1511, "stop bits (10: 1 bit)"=w1513, "flow control (0:none)"=w1515) -> ("VISA resource name out"=w1516:refnum<visa-resource-name>, "error out"=w1517:errorcluster)  [unwired: 7 in]
        n1214 = flat-sequence {
          tunnel: w1516 -> [w1519]
          tunnel: w1517 -> [w1518]
          tunnel: [w1519] -> w1509
          tunnel: [w1518] -> w1502
          frame #0 {
            n1215 = Wait (ms)(milliseconds to wait=u32 50) -> ()  [unwired: 1 out]
          }
        }
        "Residual Due" <- ""
        "Port 2 Error" <- w1502
      }
    }
    n1216 = local read "Quit"() -> (w1446:bool)
    "Error Due" <- w1451
  }
  n1217 = local write "FRICVALZ"(0.0 ("FRICVALZ")) -> ()
  n1218 = property on="RUN" class="Bool (strict)"("Visible"=TRUE) -> ()  [unwired: 2 in, 2 out]
  n1219 = while {
    tunnel: [w1536] -> _
    tunnel: [w1521] -> w54
    i -> [w1536]
    stop <- w1521 stop-if-true
    n1220 = local read "conststatus"() -> (w1525:dbl)
    n1221 = local read "Main Tab"() -> (w1523:T2)
    n1222 = local read "EDIT"() -> (w1542:bool)
    n1223 = local read "Rate"() -> (w1541:dbl)
    n1224 = case shown="True" w1542 {
      tunnel: [FALSE TRUE] -> w1528
      frame False {
      }
      frame True {
      }
    }
    n1225 = property on="Time slide" class="Slide (strict)"("Scale.Range:Maximum"=2500.0) -> ()  [unwired: 2 in, 2 out]
    n1226 = Equal?(x=w1523, y=T20."About" ("Main Tab")) -> (x = y?=w1534:bool)
    n1227 = Equal?(x=w1525, y=0.0) -> (x = y?=w1526:bool)
    n1228 = Divide(x=1.0, y=w1541) -> (x/y=w1537:dbl)
    "Time 2" <- w1537
    n1229 = case shown="True" w1526 {
      frame False {
      }
      frame True {
        # "C:\\WinDucom\\calibrate WO 2391.dcf"
        n1230 = local write "Lan flag"(22) -> ()
        n1231 = local write "conststatus"(10.0 ("rpm value : 2")) -> ()
        n1232 = String To Path(string="C:\\LAB-IQ\\calibrate WO 2465.dcf") -> (path=w1548:path)
        n1233 = Open/Create/Replace File "Open File"(file path (use dialog)=w1548) -> (refnum out=w1546:refnum<file>)  [unwired: 5 in, 2 out]
        n1234 = for {
          N: 23 -> [_]
          tunnel: w1546 -> [w1557]
          i -> [w1551]
          (unwired) TRUE ("line mode (F)")
          n1235 = Read from Text File "Read File"(file (use dialog)=w1557) -> (text=w1556:string)  [unwired: 3 in, 3 out]
          n1236 = Match Pattern(string=w1556, regular expression="]") -> (after substring=w1554:string)  [unwired: 1 in, 3 out]
          n1237 = String Subset(string=w1556, offset (0)=5, length (rest)=10 ("length (rest)")) -> (substring=w1549:string)
          n1238 = Fract/Exp String To Number(string=w1549) -> (number=w1550:dbl)  [unwired: 3 in, 1 out]
          n1239 = Match Pattern(string=w1554, regular expression="-") -> (before substring=w1552:string)  [unwired: 1 in, 3 out]
          n1240 = case shown="5" w1551 {
            tunnel: w1550 -> [w1560 w1561 w1562 w1563 _ _ _ w1568 w1569 _ w1570 w1571 w1572 w1573 w1574 w1575 _ w1576 w1577 _ _ _ _ _]
            tunnel: w1552 -> [_ _ _ _ w1564 w1565 w1566 _ _ _ _ _ _ _ _ _ _ _ _ w1578 w1579 _ w1580 _]
            frame 0 {
              n1241 = local write "FRIC. FORCE :"(w1560) -> ()
            }
            frame 1 {
              n1242 = local write "TEMPERATURE :"(w1561) -> ()
            }
            frame 2 {
              n1243 = local write "HUMIDITY:"(w1562) -> ()
            }
            frame 3 {
              n1244 = local write "AIR TEMPERATURE :"(w1563) -> ()
            }
            frame 4 {
              n1245 = local write "Com Port 1"(w1564) -> ()
            }
            frame 5 {
              n1246 = local write "Com Port 2"(w1565) -> ()
              n1247 = local write "visa due"(w1565) -> ()
            }
            frame 6 {
              n1248 = String To Path(string=w1566) -> (path=w1567:path)
              n1249 = local write "File Path"(w1567) -> ()
              "String" <- w1566
            }
            frame 7 {
              n1250 = local write "DISPLACEMENT :"(w1568) -> ()
            }
            frame 8 {
              n1251 = local write "STROKE GAIN :"(w1569) -> ()
            }
            frame 9 {
            }
            frame 10 {
              n1252 = local write "Language Selection"(w1570) -> ()
            }
            frame 11 {
              n1253 = local write "CH-POWER +"(w1571) -> ()
            }
            frame 12 {
              n1254 = local write "CH-POWER -"(w1572) -> ()
            }
            frame 13 {
              n1255 = local write "CH-HEATER"(w1573) -> ()
            }
            frame 14 {
              n1256 = local write "CH-HUMIDITY WET"(w1574) -> ()
            }
            frame 15 {
              n1257 = local write "CH-HUMIDITY DRY"(w1575) -> ()
            }
            frame 16 {
            }
            frame 17 {
              n1258 = local write "AIR TEMP INTERCEPT:"(w1576) -> ()
            }
            frame 18 {
              n1259 = local write "TEMP INTERCEPT:"(w1577) -> ()
            }
            frame 19 {
              n1260 = local write "S.NO"(w1578) -> ()
            }
            frame 20 {
              n1261 = local write "Com Port 3"(w1579) -> ()
            }
            frame 21 {
            }
            frame 22 {
              n1262 = local write "C3 :"(w1580) -> ()
            }
            frame 23, Default {
            }
          }
        }
      }
    }
    n1263 = Select(t=u32 2500 ("milliseconds to wait"), s=w1534, f=u32 500 ("milliseconds to wait")) -> (s? t:f=w1532:u32)
    n1264 = Multiply(x=w1537, y=w1532) -> (x*y=w1539:dbl)
    n1265 = property on="Time slide" class="Slide (strict)"("Visible"=w1528) -> ()  [unwired: 2 in, 2 out]
    n1266 = call "Elapsed Time2"("Time Target (s)"=w1539, "Auto Reset"=TRUE) -> ("Time has Elapsed"=w1529:bool)  [unwired: 10 in, 7 out]
    n1267 = case shown="True" w1529 {
      frame False {
      }
      frame True {
        n1268 = stacked-sequence {
          frame #0 {
            # "DATA PROCESSING"
            # "115 mV/N"
            n1269 = local read "Sample Temperature"() -> (w1581:dbl)
            "TEMP 2" <- w1581
            "TEMP 3" <- w1581
            n1270 = local read "RH Numeric:"() -> (w1588:dbl)
            n1271 = local read "HUMIDITY:"() -> (w1589:dbl)
            n1272 = local read "FRICVALZ"() -> (w1600:dbl)
            n1273 = local read "Friction"() -> (w1584:dbl)
            n1274 = local write "TEMP"(w1581) -> ()
            n1275 = Multiply(x=w1588, y=w1589) -> (x*y=→"Humidity ( %RH )" →"Hum" →"Hum 2":dbl)
            n1276 = Subtract(x=w1584, y=w1600) -> (x-y=w1595:dbl)
            "FF 2" <- w1595
            "FF 4" <- w1595
            n1277 = local read "Ambient Temperature"() -> (→"AIR TEMP":dbl)
            n1278 = local read "TEMP"() -> (w1599:dbl)
            n1279 = local write "FF 3"(w1595) -> ()
            n1280 = Compound Arithmetic op=OR("FRICVALZ 4", "FRICVALZ 3", "FRICVALZ 2") -> (w1591:bool)
            n1281 = case shown="True" w1591 {
              tunnel: w1584 -> [_ w1606]
              frame False {
              }
              frame True {
                w1605 = FALSE ("FRICVALZ")
                n1282 = local write "FRICVALZ 3"(w1605) -> ()
                n1283 = local write "FRICVALZ 2"(w1605) -> ()
                n1284 = local write "FRICVALZ 4"(w1605) -> ()
                "FRICVALZ" <- w1606
              }
            }
            n1285 = Not A Number/Path/Refnum?(number/path/refnum=w1599) -> (NaN/Path/Refnum?=w1598:bool)
            n1286 = Not A Number/Path/Refnum?(number/path/refnum=w1595) -> (NaN/Path/Refnum?=w1597:bool)
            n1287 = Divide(x=w1595, y=1.96) -> (x/y=w1592:dbl)
            n1288 = Compound Arithmetic op=OR(w1598, w1597) -> (w1596:bool)
            n1289 = Not A Number/Path/Refnum?(number/path/refnum=w1592) -> (NaN/Path/Refnum?=w1593:bool)
            n1290 = case shown="True" w1596 {
              frame False {
              }
              frame True {
                n1291 = local write "TEMP"(0.0 ("TEMP")) -> ()
